vi "K2450 Ramp.vi"() -> ()   [LabVIEW 2019]
panel:
  in  "Mode":bool
  out "Time Remaining":dbl=60.0 format="%<%H:%M:%S>t"
  out "Output Value":dbl caption="Output Voltage" format="%_4g"
  in  "Time (Hr:Min:Sec)":dbl=60.0 step=1.0 format="%<%H:%M:%S>t"
  in  "Stop Value":dbl=0.01 caption="Stop Voltage" format="%_4g"
  in  "Start Ramp":bool
  in  "Cycle Time":dbl=0.1 format="%.3g"
  in  "stop":bool
  in  "VISA resource name":refnum<visa-resource-name>
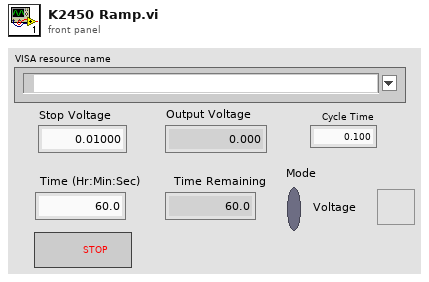
[diagram p1: front panel]
types:
  T1 = enum8{"Enabled", "Disabled", "Disabled and Grayed Out"}
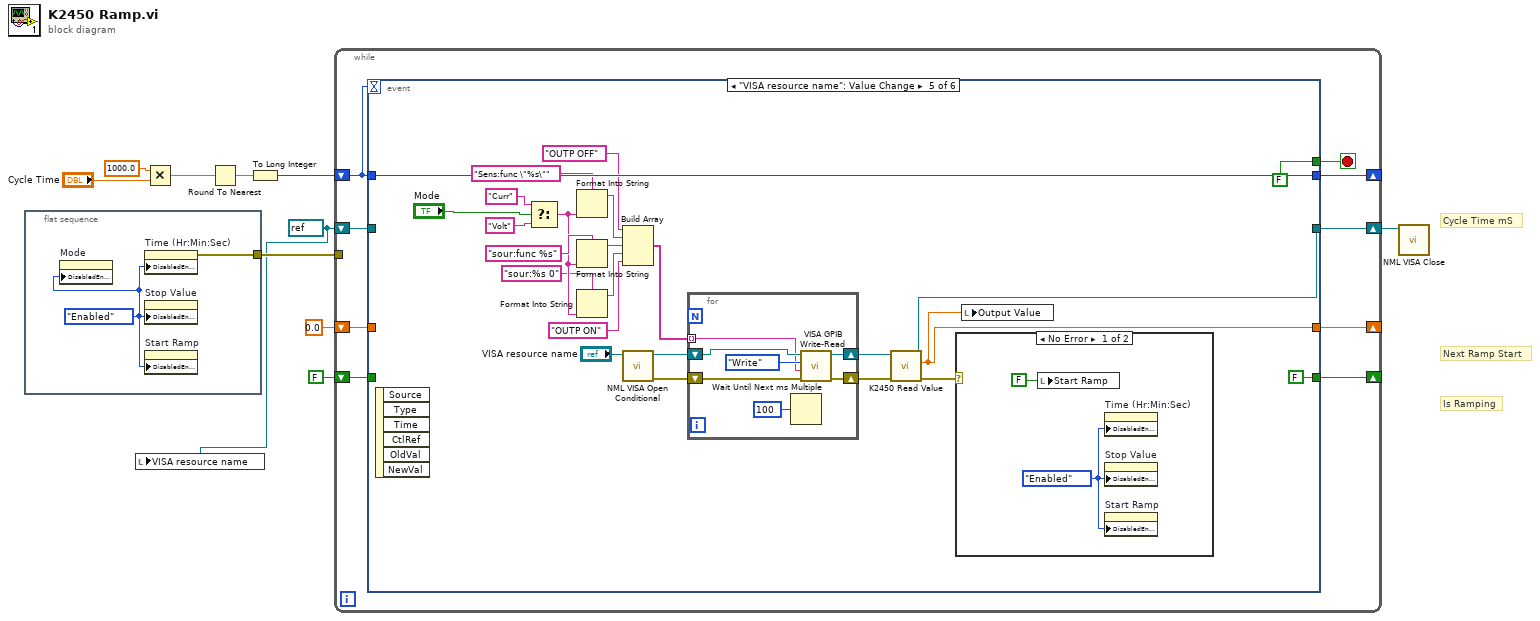
[diagram p0: block diagram]
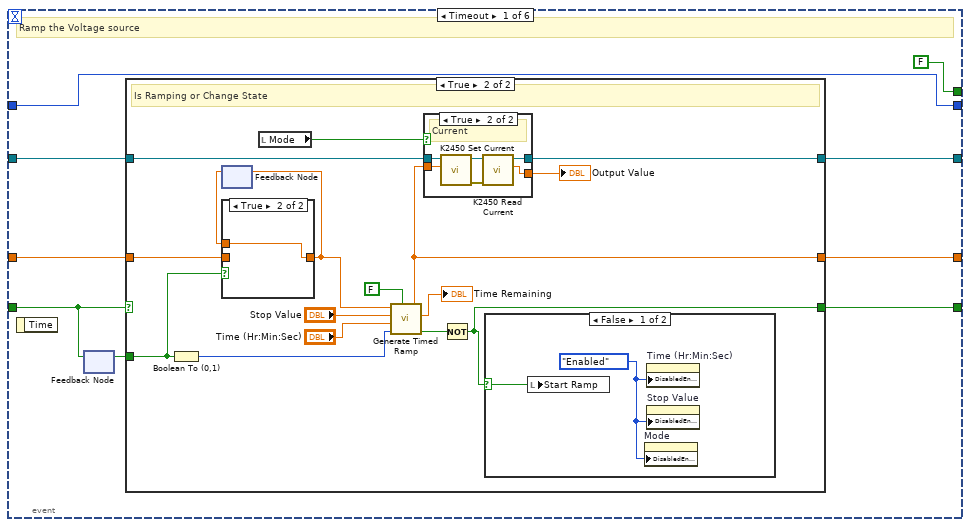
[diagram p2: hidden frame]
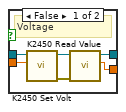
[diagram p4: hidden frame]
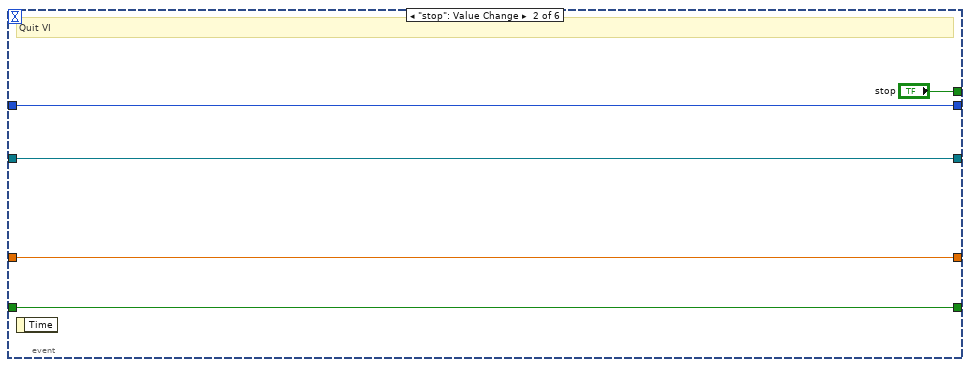
[diagram p7: hidden frame]
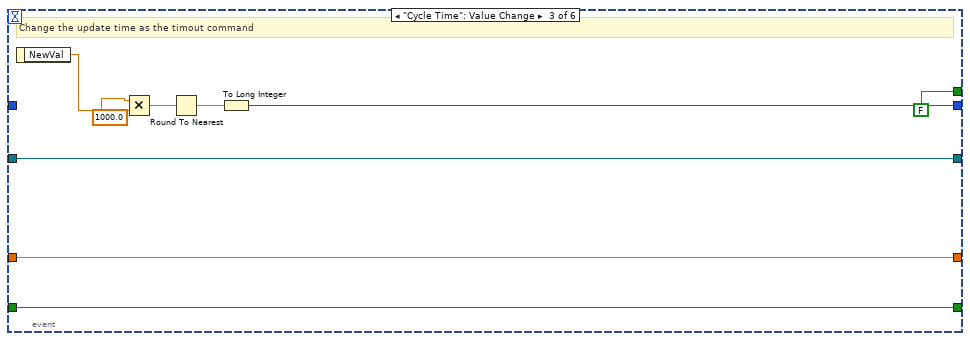
[diagram p8: hidden frame]
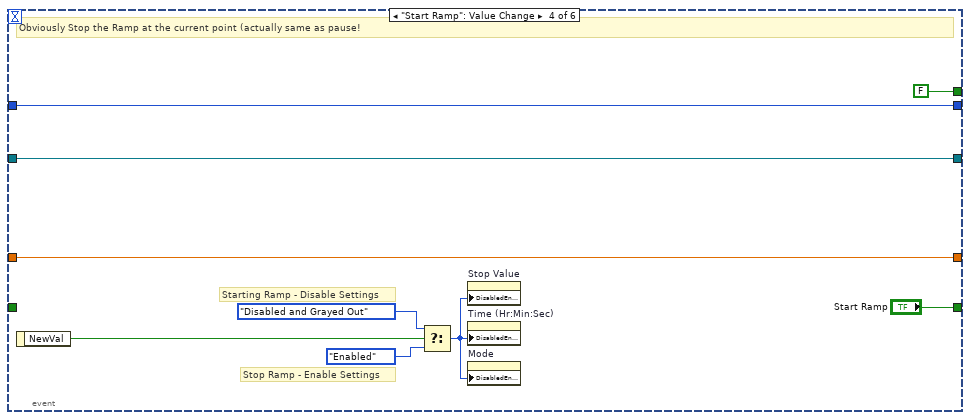
[diagram p9: hidden frame]
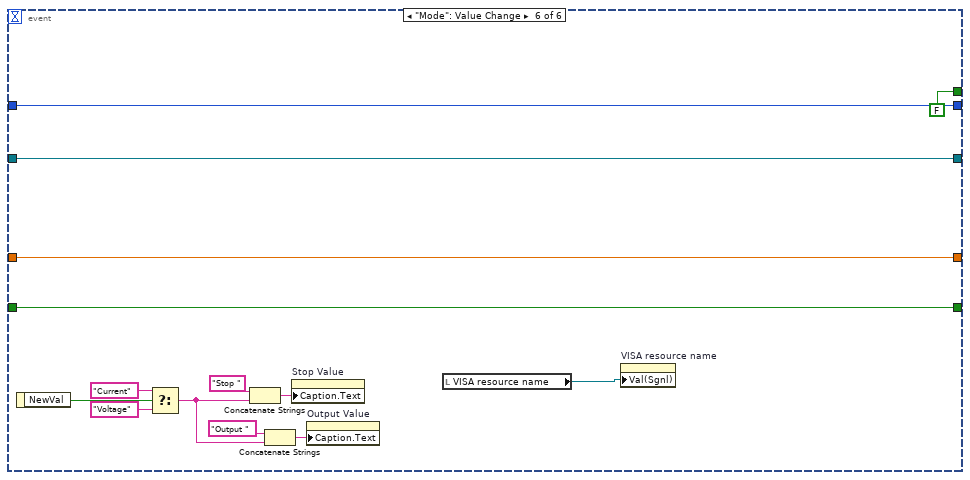
[diagram p11: hidden frame]
diagram:
  w1 = refnum<visa-resource-name> refnum ("dup VISA Session")
  # "Is Ramping"
  # "Next Ramp Start"
  # "Cycle Time mS"
  n1 = flat-sequence {
    tunnel: [w12] -> w2
    frame #0 {
      w11 = T1."Enabled" ("Disabled")
      n2 = property on="Mode" class="Bool (strict)"("DisabledEnum"=w11) -> ()  [unwired: 2 in, 2 out]
      n3 = property on="Time (Hr:Min:Sec)" class="DigNum (strict)"("DisabledEnum"=w11) -> (error out=w12:errorcluster)  [unwired: 2 in, 1 out]
      n4 = property on="Stop Value" class="DigNum (strict)"("DisabledEnum"=w11) -> ()  [unwired: 2 in, 2 out]
      n5 = property on="Start Ramp" class="Bool (strict)"("DisabledEnum"=w11) -> ()  [unwired: 2 in, 2 out]
    }
  }
  n6 = local write "VISA resource name"(w1) -> ()
  n7 = Multiply(x=1000.0, y="Cycle Time") -> (x*y=w9:dbl)
  n8 = Round To Nearest(number=w9) -> (nearest integer value=w7:dbl)
  n9 = To Long Integer(number=w7) -> (32bit integer=w6:i32)
  n10 = while {
    shift-right: [w17] -> w5
    shift-left: w1 -> [w18]
    shift-right: [w14] -> _
    shift-left: 0.0 ("Voitage 2450") -> [w13]
    shift-right: [w19] -> _
    shift-left: w6 -> [w20]
    shift-right: [w15] -> _
    shift-left: FALSE -> [w16]
    tunnel: w2 -> [_]
    stop <- w21 stop-if-true
    n11 = event shown="[4] \"VISA resource name\": Value Change" {
      selector: _ -> [_ _ _ _ _ _]
      dyn-events: _ -> [_ _ _ _ _ _]
      timeout: w20 -> [_ _ _ _ _ _]
      tunnel: [FALSE ("stop") "stop" FALSE ("stop") FALSE ("stop") FALSE ("stop") FALSE ("stop")] -> w21
      tunnel: w20 -> [w30 w69 _ w87 w106 w135]
      tunnel: [w30 w69 w75 w87 w106 w135] -> w19
      tunnel: w18 -> [w29 w66 w72 w86 _ w133]
      tunnel: [w28 w66 w72 w86 w107 w133] -> w17
      tunnel: w16 -> [w23 w68 w73 _ _ w131]
      tunnel: [w26 w68 w73 "Start Ramp" FALSE ("Start Ramp") w131] -> w15
      tunnel: [w24 w67 w71 w85 w103 w132] -> w14
      tunnel: w13 -> [w25 w67 w71 w85 _ w132]
      event Timeout {
        # "Ramp the Voltage source"
        n12 = event-data() -> ()  [unwired: 1 in, 1 out]
        n13 = feedback-in #1(w23) -> ()
        n14 = feedback #1() -> (w22:bool)  [unwired: 1 in]
        n15 = case shown="True" w23 {
          selector: w23 -> [w31 _]
          tunnel: w29 -> [w33 w48]
          tunnel: [w33 w42] -> w28
          tunnel: [w31 w40] -> w26
          tunnel: w25 -> [w32 w38]
          tunnel: [w32 w43] -> w24
          tunnel: w22 -> [_ w39]
          frame False {
            # "Idle"
          }
          frame True {
            # "Is Ramping or Change State"
            n16 = Boolean To (0,1)(Boolean=w39) -> (0, 1=w47:i16)
            n17 = feedback #2() -> (w36:dbl)  [unwired: 1 in]
            n18 = case shown="True" w39 {
              tunnel: w38 -> [w62 _]
              tunnel: [w62 w63] -> w37
              tunnel: w36 -> [_ w63]
              frame False {
              }
              frame True {
              }
            }
            n19 = feedback-in #2(w37) -> ()
            n20 = local read "Mode"() -> (w34:bool)
            n21 = call "Generate Timed Ramp.vi"("Log"=FALSE, "Point #"=w47, "Time (Hr:Min:Sec)"="Time (Hr:Min:Sec)", "Stop"="Stop Value", "Start"=w37) -> ("Stop"=w46:bool, "Time Remaining"=→"Time Remaining":dbl, "Output"=w43:dbl)  [unwired: 1 out]
            n22 = case shown="True" w34 {
              tunnel: w48 -> [w55 w58]
              tunnel: w43 -> [w54 w57]
              tunnel: [w52 w59] -> w42
              tunnel: [w51 w56] -> w41
              frame False {
                # "Voltage"
                n23 = call "K2450 Set Volt.vi"("Voltage 2450"=w54, "VISA resource name"=w55) -> ("error out"=w50:errorcluster, "dup VISA Session"=w53:refnum<visa-resource-name>)  [unwired: 8 in]
                n24 = call "K2450 Read Value.vi"("error in (no error)"=w50, "VISA resource name"=w53) -> ("Value 2450"=w51:dbl, "dup VISA Session"=w52:refnum<visa-resource-name>)  [unwired: 7 in, 1 out]
              }
              frame True {
                # "Current"
                n25 = call "K2450 Set Current.vi"("Current 2450"=w57, "VISA resource name"=w58) -> ("error out"=w61:errorcluster, "dup VISA Session"=w60:refnum<visa-resource-name>)  [unwired: 8 in]
                n26 = call "K2450 Read Current.vi"("error in (no error)"=w61, "VISA resource name"=w60) -> ("Voitage 2450"=w56:dbl, "dup VISA Session"=w59:refnum<visa-resource-name>)  [unwired: 7 in, 1 out]
              }
            }
            "Output Value" <- w41
            n27 = Not(x=w46) -> (.not. x?=w40:bool)
            n28 = case shown="False" w40 {
              selector: w40 -> [w65 _]
              frame False {
                w64 = T1."Enabled" ("Disabled")
                n29 = local write "Start Ramp"(w65) -> ()
                n30 = property on="Mode" class="Bool (strict)"("DisabledEnum"=w64) -> ()  [unwired: 2 in, 2 out]
                n31 = property on="Time (Hr:Min:Sec)" class="DigNum (strict)"("DisabledEnum"=w64) -> ()  [unwired: 2 in, 2 out]
                n32 = property on="Stop Value" class="DigNum (strict)"("DisabledEnum"=w64) -> ()  [unwired: 2 in, 2 out]
              }
              frame True {
              }
            }
          }
        }
      }
      event "stop": Value Change {
        # "Quit VI"
        n33 = event-data() -> ()  [unwired: 1 in, 1 out]
      }
      event "Cycle Time": Value Change {
        # "Change the update time as the timout command"
        n34 = event-data() -> ("NewVal"=w76:dbl)  [unwired: 1 in]
        n35 = Multiply(x=1000.0, y=w76) -> (x*y=w77:dbl)
        n36 = Round To Nearest(number=w77) -> (nearest integer value=w79:dbl)
        n37 = To Long Integer(number=w79) -> (32bit integer=w75:i32)
      }
      event "Start Ramp": Value Change {
        # "Stop Ramp - Enable Settings"
        # "Starting Ramp - Disable Settings"
        # "Obviously Stop the Ramp at the current point (actually same as pause!"
        n38 = event-data() -> ("NewVal"=w83:bool)  [unwired: 1 in]
        n39 = Select(t=T1."Disabled and Grayed Out" ("Disabled"), s=w83, f=T1."Enabled" ("Disabled")) -> (s? t:f=w80:T1)
        n40 = property on="Stop Value" class="DigNum (strict)"("DisabledEnum"=w80) -> ()  [unwired: 2 in, 2 out]
        n41 = property on="Time (Hr:Min:Sec)" class="DigNum (strict)"("DisabledEnum"=w80) -> ()  [unwired: 2 in, 2 out]
        n42 = property on="Mode" class="Bool (strict)"("DisabledEnum"=w80) -> ()  [unwired: 2 in, 2 out]
      }
      event "VISA resource name": Value Change {
        n43 = event-data() -> ()  [unwired: 1 in, 6 out]
        n44 = Select(t="Curr", s="Mode", f="Volt") -> (s? t:f=w94:string)
        n45 = Format Into String(format string="Sens:func \"%s\"", w94) -> (resulting string=w97:string)  [unwired: 2 in, 1 out]
        n46 = Format Into String(format string="sour:func %s", w94) -> (resulting string=w96:string)  [unwired: 2 in, 1 out]
        n47 = Format Into String(format string="sour:%s 0" ("initial string"), w94) -> (resulting string=w92:string)  [unwired: 2 in, 1 out]
        n48 = Build Array("OUTP OFF", w97, w96, w92, "OUTP ON") -> (w91:string[])
        n49 = call "NML VISA Open Conditional.vi"("VISA resource name"="VISA resource name") -> ("error out"=w112:errorcluster, "dup VISA Session"=w109:refnum<visa-resource-name>)  [unwired: 8 in, 1 out]
        n50 = for {
          shift-right: [w119] -> w110
          shift-left: w109 -> [w117]
          shift-right: [w120] -> w111
          shift-left: w112 -> [w118]
          tunnel: w91 -> [w116] mode=indexing
          n51 = Wait Until Next ms Multiple(millisecond multiple=u32 100) -> ()  [unwired: 1 out]
          n52 = call "VISA GPIB Write-Read.vi"("error in (no error)"=w118, "Command"=w116, "Action"=enum16{"Write", "Read", "Write & Read"}."Write", "VISA resource name"=w117) -> ("error out"=w120:errorcluster, "dup VISA Session"=w119:refnum<visa-resource-name>)  [unwired: 4 in, 2 out]
        }
        n53 = call "K2450 Read Value.vi"("error in (no error)"=w111, "VISA resource name"=w110) -> ("error out"=w104:errorcluster, "Value 2450"=w103:dbl, "dup VISA Session"=w107:refnum<visa-resource-name>)  [unwired: 7 in]
        n54 = case shown="No Error" w104 {
          frame No Error {
            w114 = T1."Enabled" ("Disabled")
            n55 = local write "Start Ramp"(FALSE ("Start Ramp")) -> ()
            n56 = property on="Time (Hr:Min:Sec)" class="DigNum (strict)"("DisabledEnum"=w114) -> ()  [unwired: 2 in, 2 out]
            n57 = property on="Stop Value" class="DigNum (strict)"("DisabledEnum"=w114) -> ()  [unwired: 2 in, 2 out]
            n58 = property on="Start Ramp" class="Bool (strict)"("DisabledEnum"=w114) -> ()  [unwired: 2 in, 2 out]
          }
          frame Error {
          }
        }
        n59 = local write "Output Value"(w103) -> ()
      }
      event "Mode": Value Change {
        n60 = event-data() -> ("NewVal"=w125:bool)  [unwired: 1 in]
        n61 = Select(t="Current" ("string"), s=w125, f="Voltage" ("string")) -> (s? t:f=w126:string)
        n62 = Concatenate Strings("Stop " ("string"), w126) -> (w128:string)
        n63 = Concatenate Strings("Output " ("string"), w126) -> (w127:string)
        n64 = property on="Stop Value" class="DigNum (strict)"("Caption.Text"=w128) -> ()  [unwired: 2 in, 2 out]
        n65 = property on="Output Value" class="DigNum (strict)"("Caption.Text"=w127) -> ()  [unwired: 2 in, 2 out]
        n66 = local read "VISA resource name"() -> (w122:refnum<visa-resource-name>)
        n67 = property on="VISA resource name" class="VISAName"("Val(Sgnl)"=w122) -> ()  [unwired: 2 in, 2 out]
      }
    }
  }
  n68 = call "NML VISA Close.vi"("VISA resource name"=w5) -> ()  [unwired: 10 in, 1 out]
